vi "GestureGloveAid.vi"() -> ()   [LabVIEW 2022 SP3]
uses:
  <vilib>/DAQmx/read.llb/DAQmx Read (Analog 1D DBL NChan 1Samp).vi
  <vilib>/DAQmx/create/channels.llb/DAQmx Create Channel (AI-Voltage-Basic).vi
  <vilib>/DAQmx/miscellaneous.llb/DAQmx Fill In Error Info.vi
panel:
  out "Numeric 5":dbl
  out "Numeric 4":dbl
  out "Numeric 3":dbl
  out "Numeric 2":dbl
  out "Numeric":dbl
  in  "physical channels":tag
  out "Waveform Chart 6":dbl(graph)
  out "Waveform Chart 5":dbl(graph)
  out "Waveform Chart 4":dbl(graph)
  out "Waveform Chart 3":dbl(graph)
  out "Waveform Chart 2":dbl[](graph)
  out "Waveform Chart":dbl(graph)
  in  "stop":bool
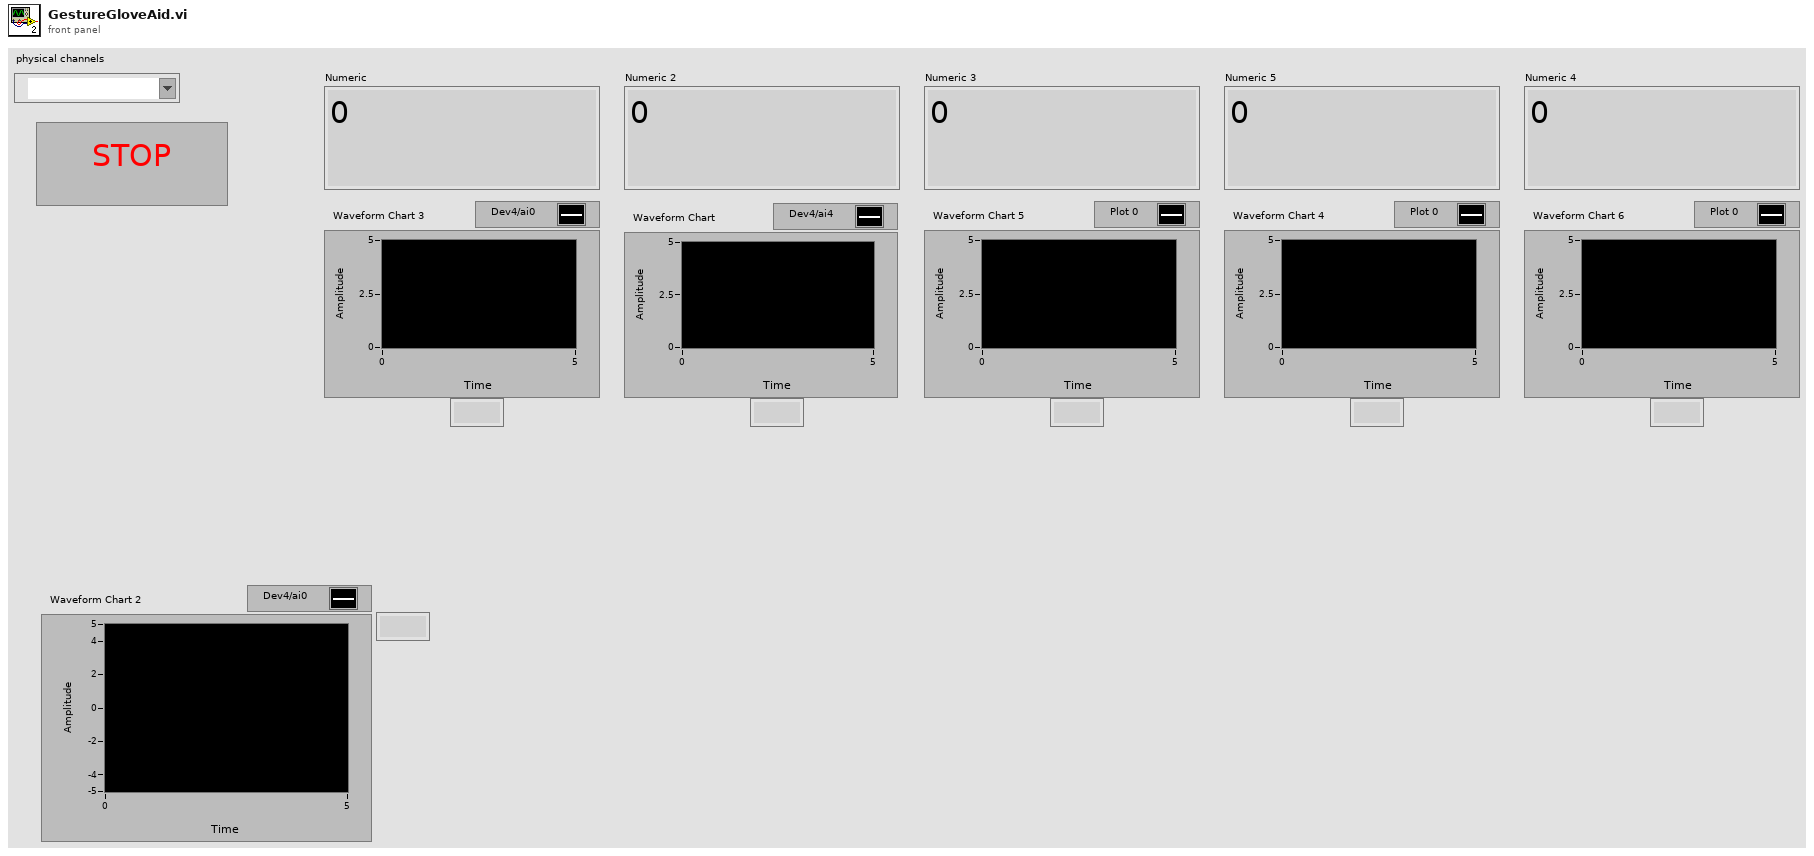
[diagram p1: front panel]
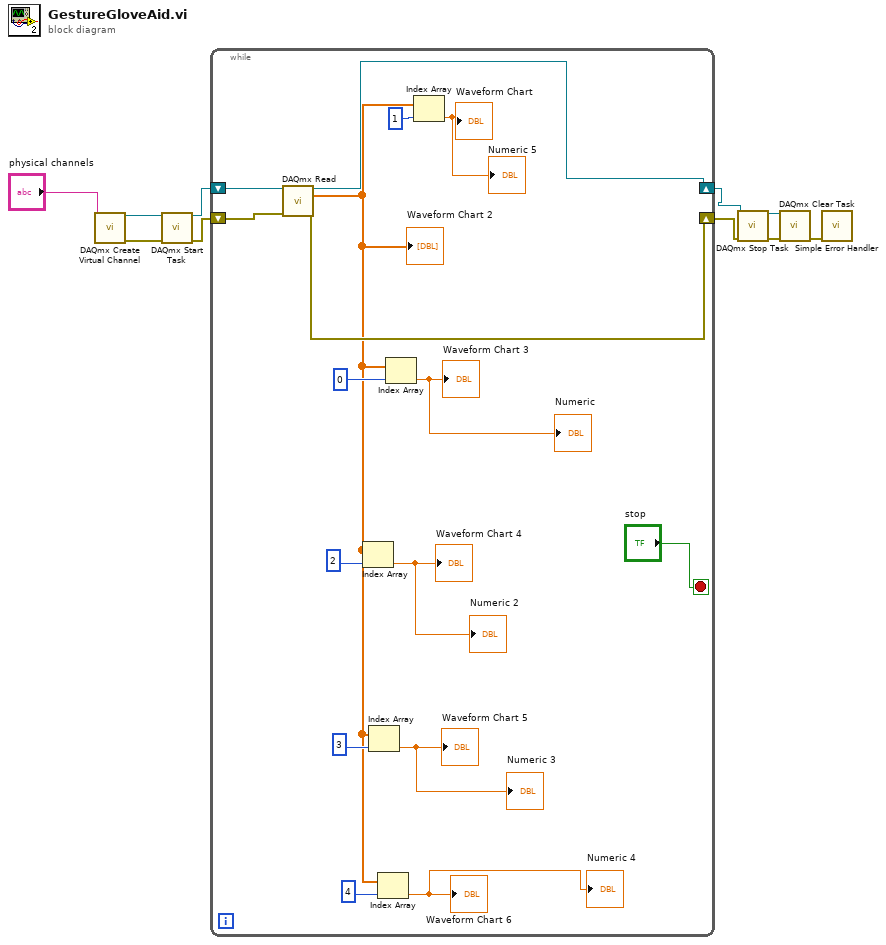
[diagram p0: block diagram]
diagram:
  n1 = call-poly <vilib>:"DAQmx Create Virtual Channel.vi"("physical channels"="physical channels") -> ("task out"=w10:refnum<k21>, "error out"=w5:errorcluster)  [unwired: 13 in]
  n2 = call <vilib>:"DAQmx Start Task.vi"("task/channels in"=w10, "error in"=w5) -> ("task out"=w9:refnum<k21>, "error out"=w4:errorcluster)  [unwired: 12 in]
  n3 = while {
    shift-right: [w25] -> w8
    shift-left: w9 -> [w26]
    shift-right: [w23] -> w3
    shift-left: w4 -> [w24]
    stop <- "stop" stop-if-true
    n4 = call-poly <vilib>:"DAQmx Read.vi"("task/channels in"=w26, "error in"=w24) -> ("task out"=w25:refnum<k21>, "data"=w16:dbl[], "error out"=w23:errorcluster)  [unwired: 11 in]
    "Waveform Chart 2" <- w16
    n5 = Index Array(array=w16, index=2 ("index (row)")) -> (element=→"Waveform Chart 4" →"Numeric 2":dbl)
    n6 = Index Array(array=w16, index=3 ("index (row)")) -> (element=→"Waveform Chart 5" →"Numeric 3":dbl)
    n7 = Index Array(array=w16, index=4 ("index (row)")) -> (element=→"Waveform Chart 6" →"Numeric 4":dbl)
    n8 = Index Array(array=w16, index=0 ("index (row)")) -> (element=→"Waveform Chart 3" →"Numeric":dbl)
    n9 = Index Array(array=w16, index=1 ("index (row)")) -> (element=→"Waveform Chart" →"Numeric 5":dbl)
  }
  n10 = call <vilib>:"DAQmx Stop Task.vi"("task/channels in"=w8, "error in"=w3) -> ("task out"=w7:refnum<k21>, "error out"=w2:errorcluster)  [unwired: 12 in]
  n11 = call <vilib>:"DAQmx Clear Task.vi"("task in"=w7, "error in"=w2) -> ("error out"=w6:errorcluster)  [unwired: 13 in]
  n12 = call <vilib>:"Simple Error Handler.vi"("error in (no error)"=w6) -> ()  [unwired: 4 in, 5 out]
